vi "Timestamp.vi"() -> ()   [LabVIEW 2018]
doc: "This example performs a serial port write and a serial port read. The parameters set for the serial port must match the parameters of the connected instrument or device. The VISA Configure Serial Port VI sets the configuration parameters. The front panel displays the controls used to configure the basic parameters, such as baud rate, data bits, and parity. The VI passes the VISA resource name to other VIs that perform operations on that VISA resource. The VISA Write function sends a command to the serial device and the VISA Read function returns data based on the command. The VISA Close function then closes the reference to the serial device. It is important to close the reference; otherwise, further communication through that port might not be possible."
uses:
  <vilib>/Instr/_visa.llb/VISA Configure Serial Port (Instr).vi
  <vilib>/Utility/file.llb/Write Delimited Spreadsheet (I64).vi
panel:
  out "Write Status":string="No save path defined!"
  in  "Gate Time":dbl=300.0
  in  "TTL/NIM Box":string(combo)="TTL;"
  in  "Save Timestamp of <<LAST LOOP>> in File After STOP":path
  out "Byte Array of All Loops":i32[][](array[numeric])
  out "output array":u32[][](array[numeric])
  out "spreadsheet string":string
  out "Current Byte Array":u8[](array[numeric])
  in  "stop":bool
  in  "Serial Settings":T1={"baud rate"=115200, "data bits"=8, "parity"=enum."None", "stop bits"=10, "flow control"=2} {"flow control" items=["None"=0, "XON/XOFF"=1, "RTS/CTS"=2, "DTR/DSR"=4]; "stop bits" items=["1.0"=10, "1.5"=15, "2.0"=20]; "data bits" min=5 max=8 step=1; "baud rate" items=["75"=75, "110"=110, "134"=134, "150"=150, "300"=300, "600"=600, "1200"=1200, "1800"=1800, "2400"=2400, "4800"=4800, "7200"=7200, "4"=9600, "14400"=14400, "19200"=19200, "28800"=28800, "38400"=38400, "56000"=56000, "57600"=57600, "115200"=115200, "128000"=128000, "230400"=230400]}
  in  "VISA resource name":refnum<visa-resource-name>="COM1"
  # "Overview: Demonstrates the use of NI-VISA for reading USB Time Stamp Counter.  The commands for device is in Wiki. In this VI , termination characters are not used because they do not exist in the return message. The 27-bit timestamp values are converted to 32bit long integers then multiplied by 2 ns, the long number in the spreadsheet string is timestamp in [ns].\nString Format:\n[No Counts (1/0)] [Channel 4 Event (1/0)] [Channel 3 Event (1/0)] [Channel 2 Event (1/0)]  [Channel 1 Event (1/0)] [32-bit long timestamp [ns]]"
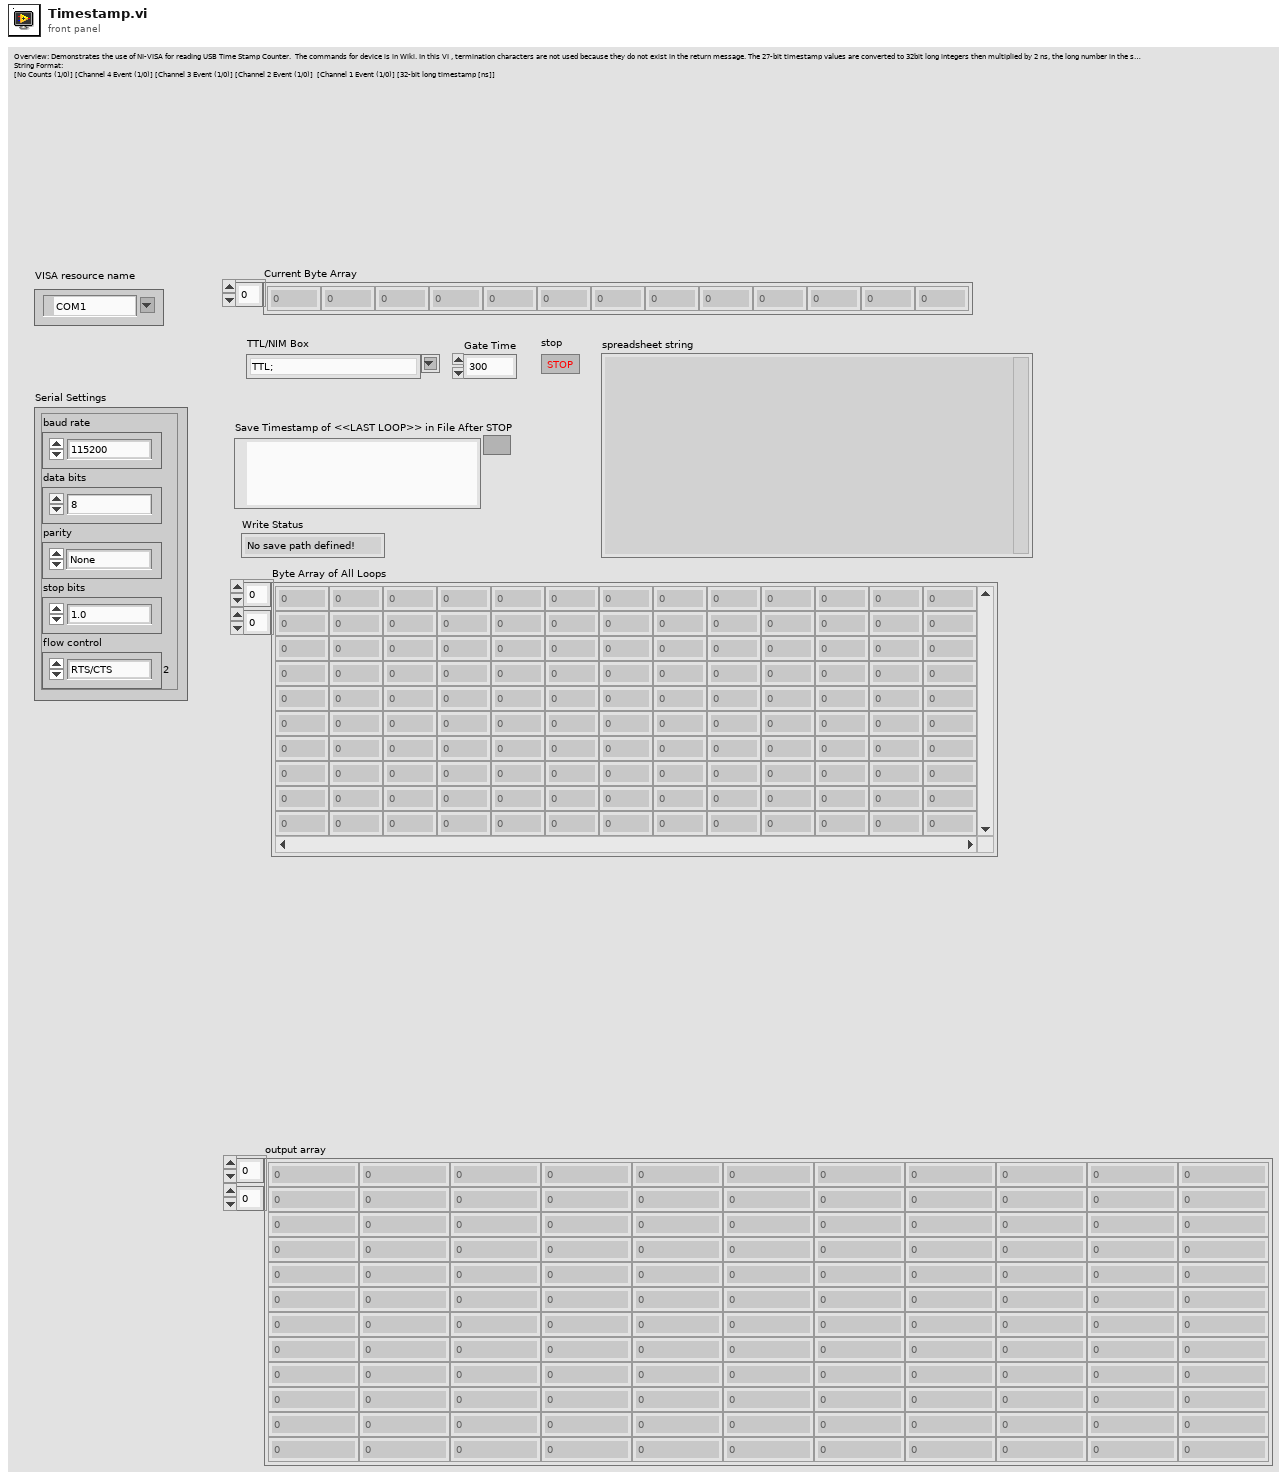
[diagram p1: front panel]
types:
  T1 = cluster{"baud rate":u32, "data bits":u16, "parity":enum16{"None", "Odd", "Even", "Mark", "Space"}, "stop bits":u16, "flow control":u16}
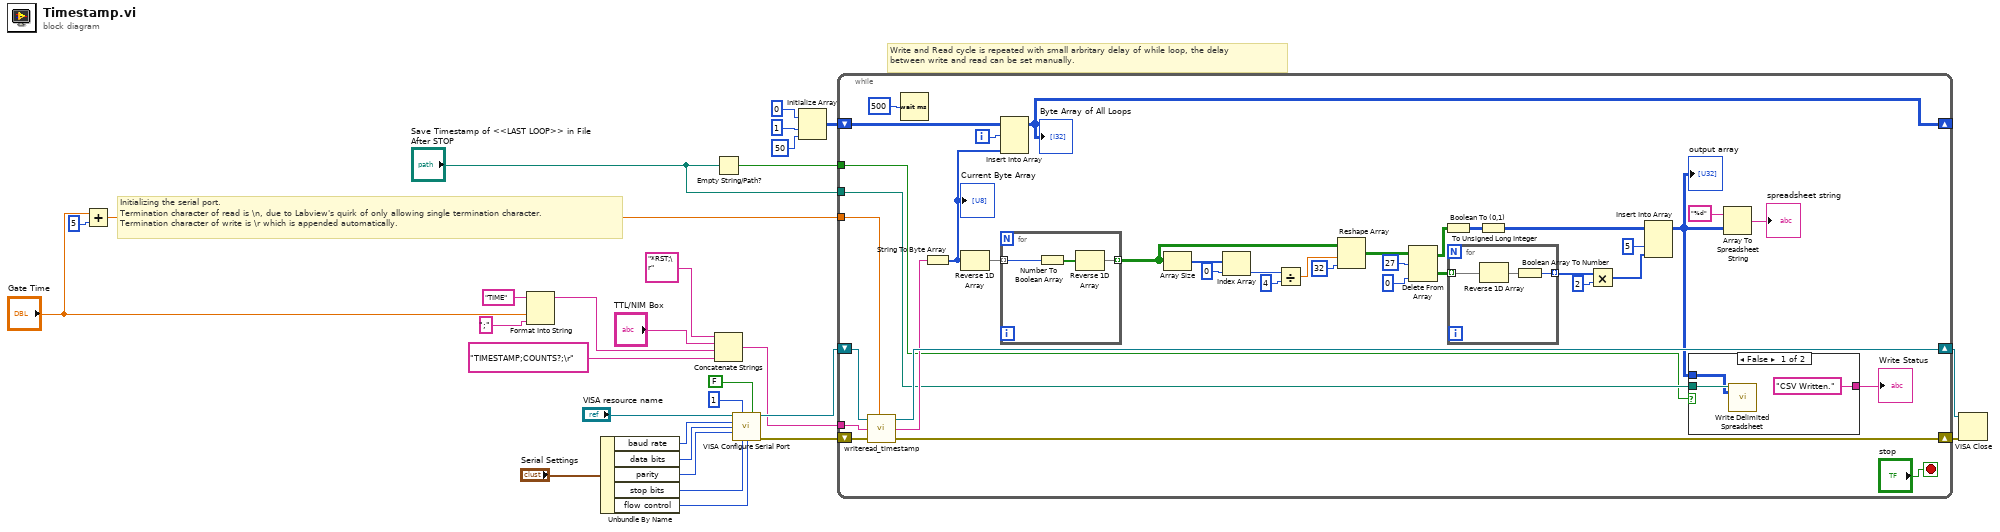
[diagram p0: block diagram]
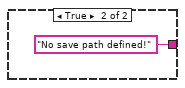
[diagram p2: hidden frame]
diagram:
  # "Write and Read cycle is repeated with small arbritary delay of while loop, the delay \nbetween write and read can be set manually."
  # "Initializing the serial port.\nTermination character of read is \\n, due to Labview's quirk of only allowing single termination character.\nTermination character of write is \\r which is appended automatically."
  n1 = Add(x="Gate Time", y=5) -> (x+y=w3:dbl)
  n2 = Format Into String(initial string="TIME", "Gate Time", ";") -> (resulting string=w7:string)  [unwired: 2 in, 1 out]
  n3 = Unbundle By Name("Serial Settings") -> ("baud rate"=w27:u32, "data bits"=w26:u16, "parity"=w25:enum16{"None", "Odd", "Even", "Mark", "Space"}, "stop bits"=w24:u16, "flow control"=w23:u16)
  n4 = Empty String/Path?(string/path="Save Timestamp of <<LAST LOOP>> in File After STOP") -> (empty?=w1:bool)
  n5 = Concatenate Strings("*RST;\r" ("Command (*RST;TTL;TIME200;TIMESTAMP;COUNTS?;)"), "TTL/NIM Box", w7, "TIMESTAMP;COUNTS?;\r" ("Command (*RST;TTL;TIME200;TIMESTAMP;COUNTS?;)")) -> (w10:string)
  n6 = call-poly "VISA Configure Serial Port"("VISA resource name"="VISA resource name", "timeout (10sec)"=1, "Enable Termination\nChar (T)"=FALSE, "baud rate (9600)"=w27, "data bits (8)"=w26, "parity (0:none)"=w25, "stop bits (10: 1 bit)"=w24, "flow control (0:none)"=w23) -> ("VISA resource name out"=w19:refnum<visa-resource-name>, "error out"=w13:errorcluster)  [unwired: 1 in, 5 out]
  n7 = Initialize Array(0, 1, 50) -> (w16:i32[][])
  n8 = while {
    tunnel: w3 -> [w63]
    tunnel: w10 -> [w60]
    shift-right: [w57] -> w20
    shift-left: w13 -> [w59]
    shift-right: [w61] -> w21
    shift-left: w19 -> [w62]
    shift-right: [w64] -> _
    shift-left: w16 -> [w66]
    tunnel: "Save Timestamp of <<LAST LOOP>> in File After STOP" -> [w34]
    tunnel: w1 -> [w31]
    i -> [w65]
    stop <- "stop" stop-if-true
    n9 = call "writeread_timestamp.vi"("VISA resource input"=w62, "Read Delay"=w63, "write buffer"=w60, "error in (no error)"=w59) -> ("VISA resource out"=w61:refnum<visa-resource-name>, "Response 2"=w58:string, "error out"=w57:errorcluster)  [unwired: 3 in]
    n10 = Wait (ms)(milliseconds to wait=500) -> ()  [unwired: 1 out]
    n11 = String To Byte Array(string=w58) -> (unsigned byte array=w55:u8[])
    "Current Byte Array" <- w55
    n12 = Reverse 1D Array(array=w55) -> (reversed array=w54:u8[])
    n13 = Insert Into Array(array=w66, index (row)=w65, new element=w55) -> (w64:i32[][])  [unwired: 1 in]
    "Byte Array of All Loops" <- w64
    n14 = for {
      tunnel: w54 -> [w77] mode=indexing
      tunnel: [w75] -> w49 mode=indexing
      n15 = Number To Boolean Array(number=w77) -> (Boolean array=w76:bool[])
      n16 = Reverse 1D Array(array=w76) -> (reversed array=w75:bool[])
    }
    n17 = Array Size(array=w49) -> (size(s)=w52:i32[])
    n18 = Index Array(array=w52, index=0) -> (element=w50:i32)
    n19 = Divide(x=w50, y=4) -> (x/y=w48:dbl)
    n20 = Reshape Array(w49, w48, 32) -> (w46:bool[][])
    n21 = Delete From Array(array=w46, length=27, index (col)=0) -> (deleted portion=w43:bool[][], array with subset deleted=w42:bool[][])  [unwired: 1 in]
    n22 = Boolean To (0,1)(Boolean=w42) -> (0, 1=w39:i16[][])
    n23 = for {
      tunnel: w43 -> [w73] mode=indexing
      tunnel: [w74] -> w36 mode=indexing
      n24 = Reverse 1D Array(array=w73) -> (reversed array=w72:bool[])
      n25 = Boolean Array To Number(Boolean array=w72) -> (number=w74:u32)
    }
    n26 = To Unsigned Long Integer(number=w39) -> (unsigned 32bit integer=w38:u32[][])
    n27 = Multiply(x=w36, y=2) -> (x*y=w35:u32[])
    n28 = Insert Into Array(array=w38, index (col)=5, new element=w35) -> (w32:u32[][])  [unwired: 1 in]
    "output array" <- w32
    n29 = case shown="False" w31 {
      tunnel: w34 -> [w70 _]
      tunnel: w32 -> [w69 _]
      tunnel: ["CSV Written." "No save path defined!"] -> w30
      frame False {
        n30 = call-poly <vilib>:"Write Delimited Spreadsheet.vi"("file path (dialog if empty)"=w70, "2D data"=w69) -> ()  [unwired: 12 in, 2 out]
      }
      frame True {
      }
    }
    "Write Status" <- w30
    n31 = Array To Spreadsheet String(array=w32, 3:"%d") -> (spreadsheet string=→"spreadsheet string":string)  [unwired: 1 in]
  }
  n32 = VISA Close(VISA resource name=w21, error in (no error)=w20) -> ()  [unwired: 1 out]
